vi "PrepData.vi"(0 "object in":refnum<class "TDMSLogger.lvclass">, 1 "Elapsed Time":dbl, 2 "ChannelsWFIn":waveform(dbl)[](array[waveform]), 3 "AmplitudeAndVoltageSettings":T4, 4 "MeTecData":T3={"meTEC_CH2_Temperature Stability"=1, "meTEC_CH2_Act. Output Current [A]"=0.0, "meTEC_CH2_Act. Output Voltage [V]"=0.0, "meTEC_CH2_Object Temperature [°C]"=0.0, "meTEC_CH2_Sink Temperature [°C]"=0.0, "meTEC_CH1_Error Parameter"=0, "meTEC_CH1_Error Instance"=0, "meTEC_CH1_Error No."=0, "meTEC_CH1_Device Status"=1, "meTEC_CH1_Temperature Stability"=1, "meTEC_CH1_Act. Output Current [A]"=0.0, "meTEC_CH1_Act. Output Voltage [V]"=0.0, "meTEC_CH1_Object Temperature [°C]"=0.0, "meTEC_CH1_Sink Temperature [°C]"=0.0} {"meTEC_CH1_Sink Temperature [°C]" format="%.3f"; "meTEC_CH1_Object Temperature [°C]" format="%.3f"; "meTEC_CH1_Act. Output Voltage [V]" format="%.3f"; "meTEC_CH1_Act. Output Current [A]" format="%.3f"; "meTEC_CH1_Temperature Stability" items=["Temperature regulation is not active", "Is not stable", "Is stable"]; "meTEC_CH1_Device Status" items=["Initializing", "Ready", "Run", "Error", "Bootloader", "Reset in Progress"]; "meTEC_CH2_Sink Temperature [°C]" format="%.3f"; "meTEC_CH2_Object Temperature [°C]" format="%.3f"; "meTEC_CH2_Act. Output Voltage [V]" format="%.3f"; "meTEC_CH2_Act. Output Current [A]" format="%.3f"; "meTEC_CH2_Temperature Stability" items=["Temperature regulation is not active", "Is not stable", "Is stable"]}, 5 "error in (no error)":errorcluster, 6 "AGTemp":dbl, 7 "SetPower":dbl, 8 "MCC TempData":dbl[](array[numeric]), 9 "MeasuredPower":dbl, 11 "AmplitudeOk":bool, 13 "WfgEnabled":cluster{"Ch1":bool, "Ch2":bool}) -> (14 "object out":refnum<class "TDMSLogger.lvclass">, 16 "Channel Names":string[](array[string]), 17 "Channels(WF)":waveform(dbl)[](array[waveform]), 19 "error out":errorcluster)   [LabVIEW 2019, in "TDMSLogger.lvclass"]
uses:
  TDMSLogger.lvclass
  TEC LabVIEW Control Software v0.14/Source/LV Source/[meerstetter engineering TE Cooling]/TypeDefs/meTEC_ID 1200_Temperature is Stable.ctl
  TEC LabVIEW Control Software v0.14/Source/LV Source/[meerstetter engineering TE Cooling]/TypeDefs/meTEC_ID 104_Device Status.ctl
  <vilib>/measure/matone.llb/Extract Single Tone Information 1 Chan.vi
  <vilib>/measure/NI_MAPro.lvlib
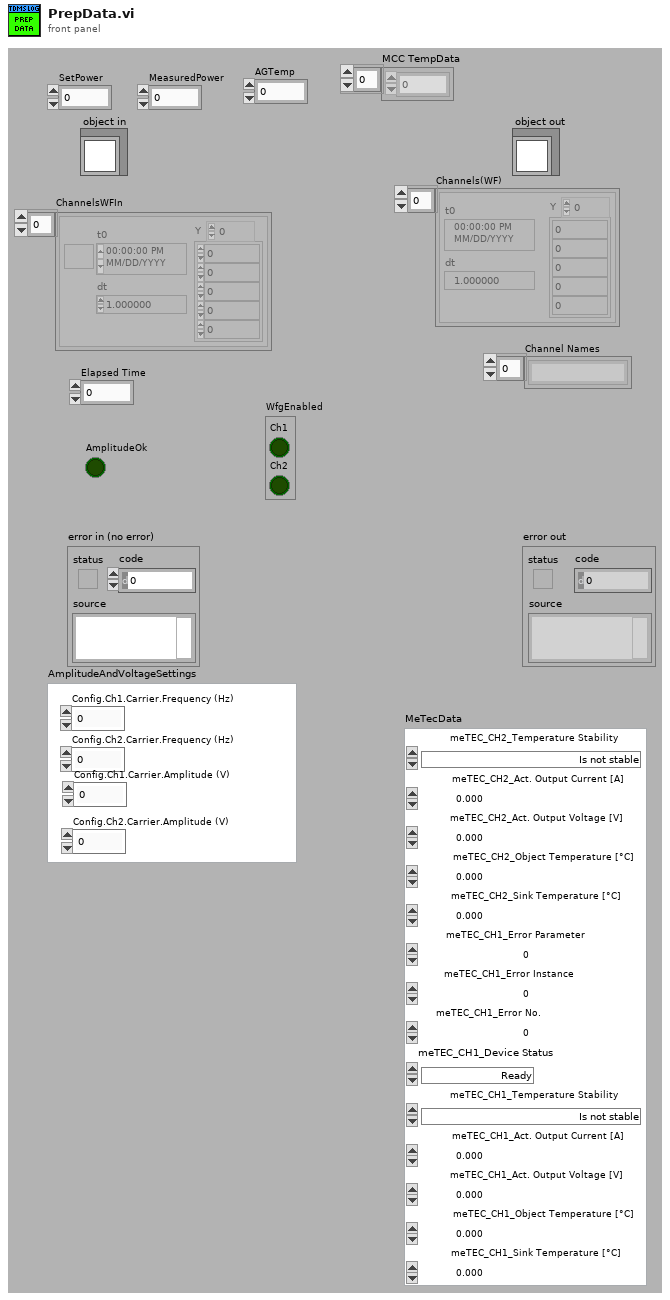
[diagram p1: front panel]
types:
  T1 = typedef "meTEC_ID 1200_Temperature is Stable.ctl" = i32
  T2 = typedef "meTEC_ID 104_Device Status.ctl" = i32
  T3 = cluster{"meTEC_CH2_Temperature Stability":T1, "meTEC_CH2_Act. Output Current [A]":dbl, "meTEC_CH2_Act. Output Voltage [V]":dbl, "meTEC_CH2_Object Temperature [°C]":dbl, "meTEC_CH2_Sink Temperature [°C]":dbl, "meTEC_CH1_Error Parameter":i32, "meTEC_CH1_Error Instance":i32, "meTEC_CH1_Error No.":i32, "meTEC_CH1_Device Status":T2, "meTEC_CH1_Temperature Stability":T1, "meTEC_CH1_Act. Output Current [A]":dbl, "meTEC_CH1_Act. Output Voltage [V]":dbl, "meTEC_CH1_Object Temperature [°C]":dbl, "meTEC_CH1_Sink Temperature [°C]":dbl}
  T4 = cluster{"Config.Ch1.Carrier.Frequency (Hz)":dbl, "Config.Ch2.Carrier.Frequency (Hz)":dbl, "Config.Ch1.Carrier.Amplitude (V)":dbl, "Config.Ch2.Carrier.Amplitude (V)":dbl}
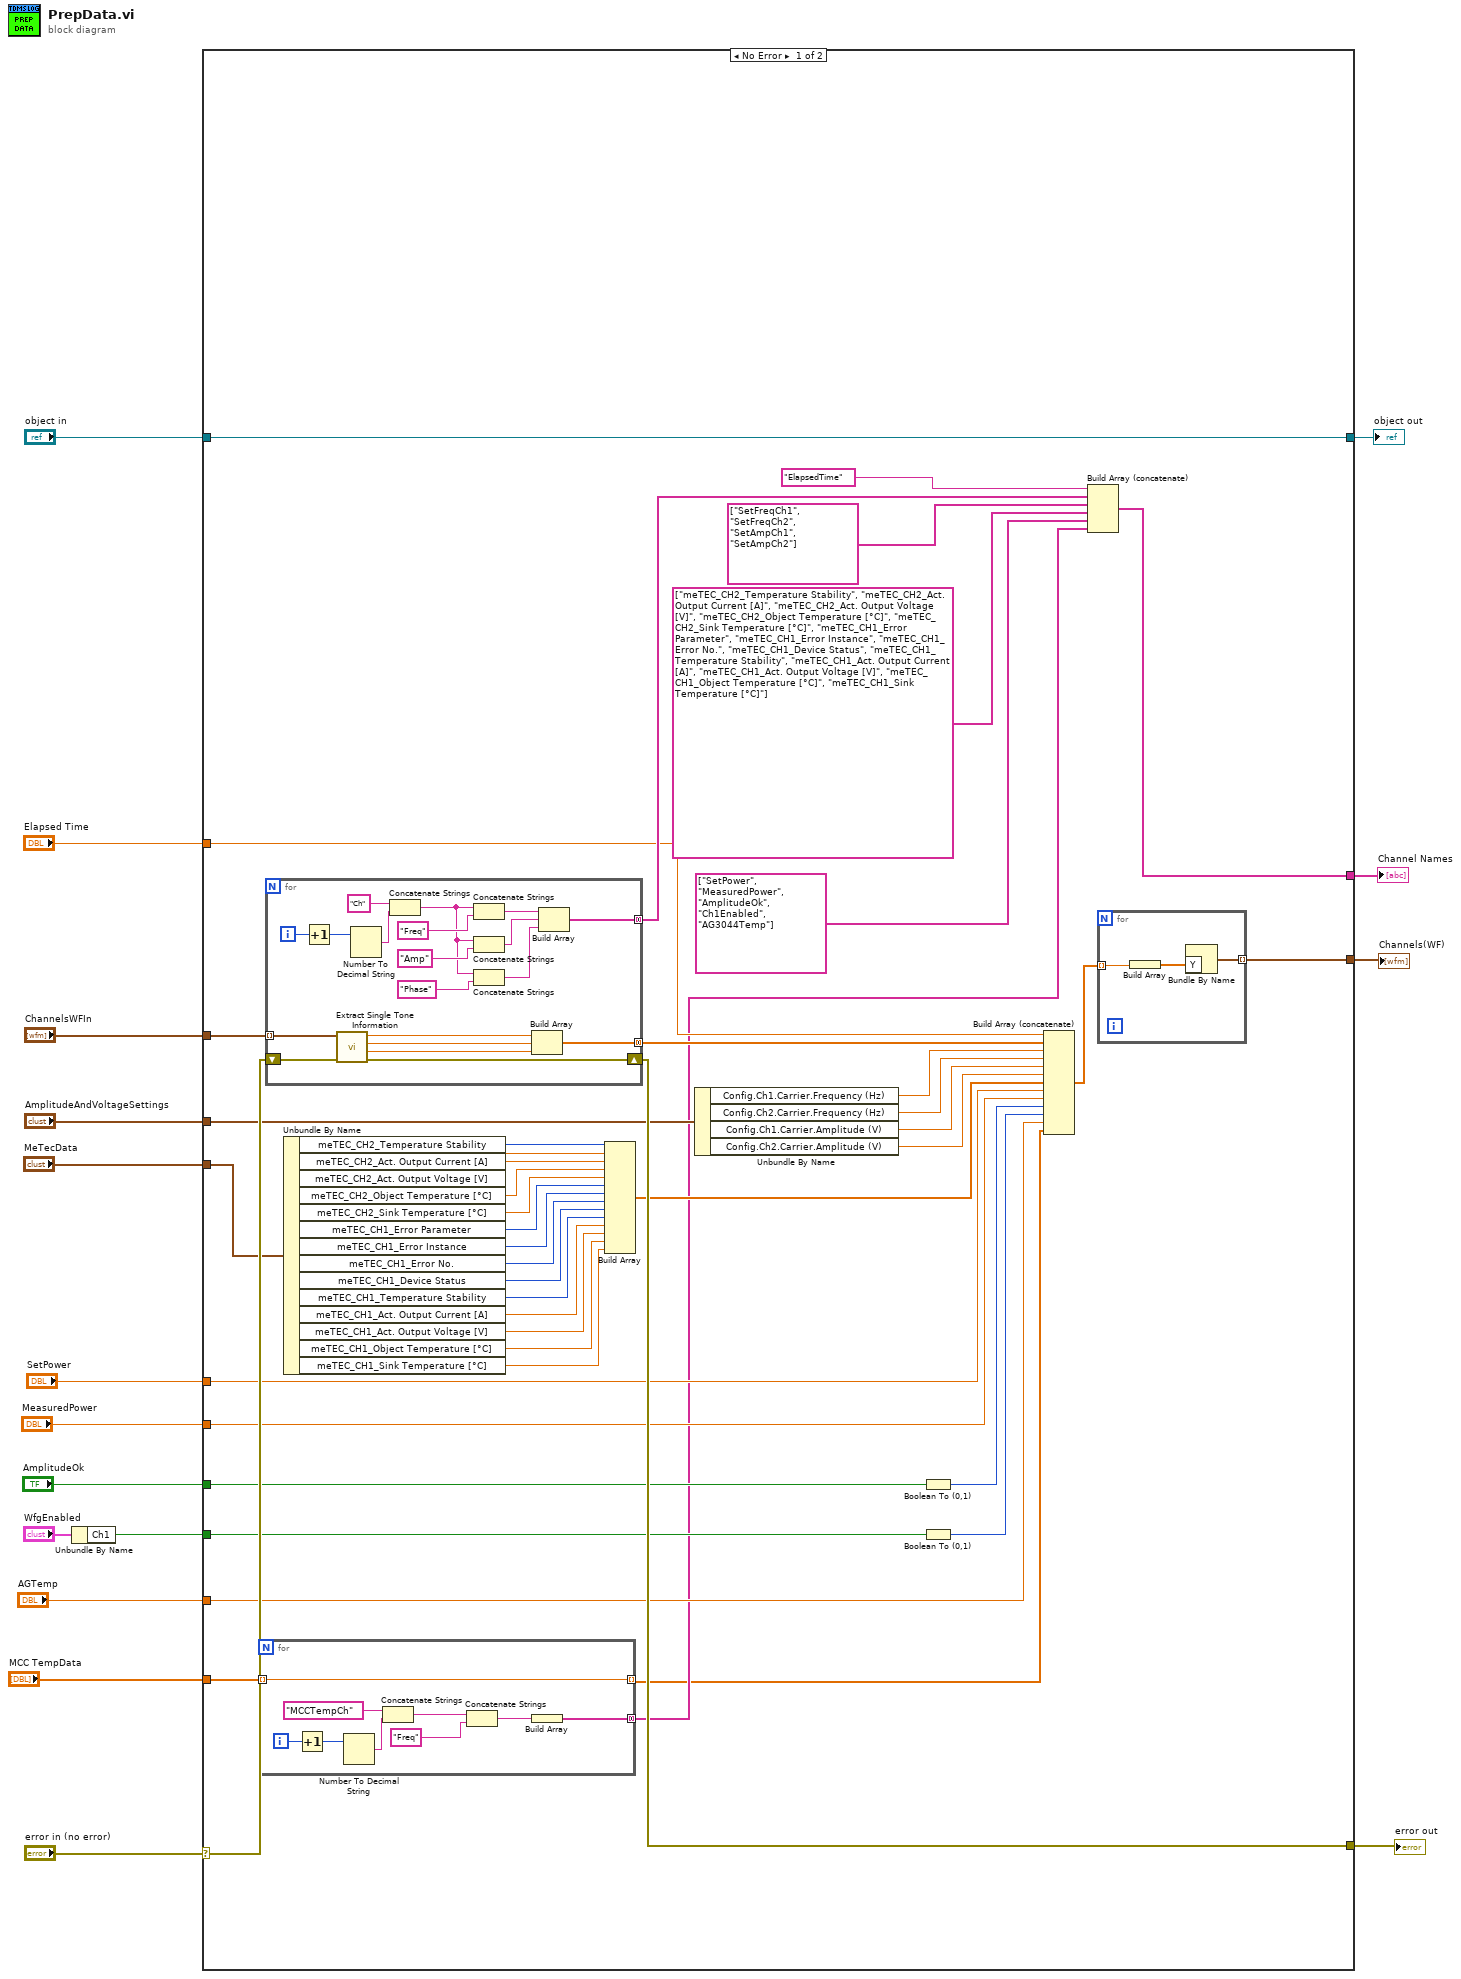
[diagram p0: block diagram]
diagram:
  n1 = Unbundle By Name("WfgEnabled") -> ("Ch1"=w3:bool)
  n2 = case shown="No Error" "error in (no error)" {
    selector: "error in (no error)" -> [w52 w95]
    tunnel: [w51 w95] -> w16
    tunnel: [w62 w94] -> w14
    tunnel: "object in" -> [w62 w94]
    tunnel: [w60 _] -> w13
    tunnel: [w56 _] -> w12
    tunnel: "AmplitudeAndVoltageSettings" -> [w34 _]
    tunnel: "ChannelsWFIn" -> [w54 _]
    tunnel: "MeTecData" -> [w48 _]
    tunnel: "Elapsed Time" -> [w31 _]
    tunnel: "SetPower" -> [w28 _]
    tunnel: "MeasuredPower" -> [w27 _]
    tunnel: "AmplitudeOk" -> [w25 _]
    tunnel: w3 -> [w23 _]
    tunnel: "AGTemp" -> [w21 _]
    tunnel: "MCC TempData" -> [w19 _]
    frame No Error {
      n3 = for {
        tunnel: [w65] -> w20 mode=concatenating
        tunnel: w19 -> [w63] mode=indexing
        tunnel: [w63] -> w18 mode=indexing
        i -> [w69]
        n4 = Increment(x=w69) -> (x+1=w66:i32)
        n5 = Number To Decimal String(number=w66) -> (decimal integer string=w70:string)  [unwired: 1 in]
        n6 = Concatenate Strings("MCCTempCh" ("string"), w70) -> (w64:string)
        n7 = Concatenate Strings(w64, "Freq") -> (w67:string)
        n8 = Build Array(w67) -> (w65:string[])
      }
      n9 = for {
        tunnel: [w85] -> w55 mode=concatenating
        shift-right: [w80] -> w51
        shift-left: w52 -> [w81]
        tunnel: [w76] -> w53 mode=concatenating
        tunnel: w54 -> [w75] mode=indexing
        i -> [w91]
        n10 = Increment(x=w91) -> (x+1=w86:i32)
        n11 = call-poly <vilib>:"Extract Single Tone Information.vi"("error in (no error)"=w81, "time signal in"=w75) -> ("error out"=w80:errorcluster, "detected phase (deg)"=w77:dbl, "detected amplitude"=w78:dbl, "detected frequency"=w79:dbl)  [unwired: 4 in, 2 out]
        n12 = Number To Decimal String(number=w86) -> (decimal integer string=w92:string)  [unwired: 1 in]
        n13 = Concatenate Strings("Ch" ("string"), w92) -> (w84:string)
        n14 = Concatenate Strings(w84, "Freq") -> (w88:string)
        n15 = Concatenate Strings(w84, "Amp") -> (w87:string)
        n16 = Concatenate Strings(w84, "Phase") -> (w82:string)
        n17 = Build Array(w79, w78, w77) -> (w76:dbl[])
        n18 = Build Array(w88, w87, w82) -> (w85:string[])
      }
      n19 = Unbundle By Name(w48) -> ("meTEC_CH2_Temperature Stability"=w47:T1, "meTEC_CH2_Act. Output Current [A]"=w46:dbl, "meTEC_CH2_Act. Output Voltage [V]"=w45:dbl, "meTEC_CH2_Object Temperature [°C]"=w44:dbl, "meTEC_CH2_Sink Temperature [°C]"=w43:dbl, "meTEC_CH1_Error Parameter"=w42:i32, "meTEC_CH1_Error Instance"=w41:i32, "meTEC_CH1_Error No."=w40:i32, "meTEC_CH1_Device Status"=w39:T2, "meTEC_CH1_Temperature Stability"=w38:T1, "meTEC_CH1_Act. Output Current [A]"=w37:dbl, "meTEC_CH1_Act. Output Voltage [V]"=w36:dbl, "meTEC_CH1_Object Temperature [°C]"=w35:dbl, "meTEC_CH1_Sink Temperature [°C]"=w26:dbl)
      n20 = Build Array(w47, w46, w45, w44, w43, w42, w41, w40, w39, w38, w37, w36, w35, w26) -> (w33:dbl[])
      n21 = Unbundle By Name(w34) -> ("Config.Ch1.Carrier.Frequency (Hz)"=w59:dbl, "Config.Ch2.Carrier.Frequency (Hz)"=w58:dbl, "Config.Ch1.Carrier.Amplitude (V)"=w50:dbl, "Config.Ch2.Carrier.Amplitude (V)"=w49:dbl)
      n22 = Boolean To (0,1)(Boolean=w25) -> (0, 1=w24:i16)
      n23 = Boolean To (0,1)(Boolean=w23) -> (0, 1=w22:i16)
      n24 = Build Array (concatenate)(w31, w53, w59, w58, w50, w49, w33, w28, w27, w24, w22, w21, w18) -> (w61:dbl[])
      n25 = Build Array (concatenate)("ElapsedTime", w55, string[] ["SetFreqCh1", "SetFreqCh2", "SetAmpCh1", "SetAmpCh2"] ("channel name(s) in (Untitled)"), string[] ["meTEC_CH2_Temperature Stability", "meTEC_CH2_Act. Output Current [A]", "meTEC_CH2_Act. Output Voltage [V]", "meTEC_CH2_Object Temperature [°C]", "meTEC_CH2_Sink Temperature [°C]", "meTEC_CH1_Error Parameter", "meTEC_CH1_Error Instance", "meTEC_CH1_Error No.", "meTEC_CH1_Device Status", "meTEC_CH1_Temperature Stability", "meTEC_CH1_Act. Output Current [A]", "meTEC_CH1_Act. Output Voltage [V]", "meTEC_CH1_Object Temperature [°C]", "meTEC_CH1_Sink Temperature [°C]"] ("Array"), string[] ["SetPower", "MeasuredPower", "AmplitudeOk", "Ch1Enabled", "AG3044Temp"] ("channel name(s) in (Untitled)"), w20) -> (w56:string[])
      n26 = for {
        tunnel: w61 -> [w74] mode=indexing
        tunnel: [w72] -> w60 mode=indexing
        n27 = Build Array(w74) -> (w73:dbl[])
        n28 = Bundle By Name("Y"=w73) -> (w72:waveform(dbl))  [unwired: 1 in]
      }
    }
    frame Error {
    }
  }
  "error out" <- w16
  "object out" <- w14
  "Channels(WF)" <- w13
  "Channel Names" <- w12
